vi "test_CCDSetAndGetGain.vi"   [LabVIEW 2023]
uses:
  <vilib>/JDP Science/JSONtext/Variant to JSON Text.vi
  <vilib>/JDP Science/JSONtext/Set Item.vi
  <vilib>/JDP Science/JSONtext/LVClass Serializer/JSONtext LVClass Serializer.lvclass
  Source/Classes/CCD/CCD.lvclass
  <vilib>/addons/_JKI Toolkits/Caraya/classes/Assert/Assert.lvclass
  <vilib>/addons/_JKI Toolkits/Caraya/classes/Test/Test.lvclass
  <vilib>/addons/_JKI Toolkits/Caraya/classes/Assert/Assert Equal Value and Type_Variant.vi
  <vilib>/addons/_JKI Toolkits/Caraya/classes/Assert/Assert Not Error.vi
types:
  T1 = enum16{"High Light", "Best Dynamic Range", "High Sensitivity"}
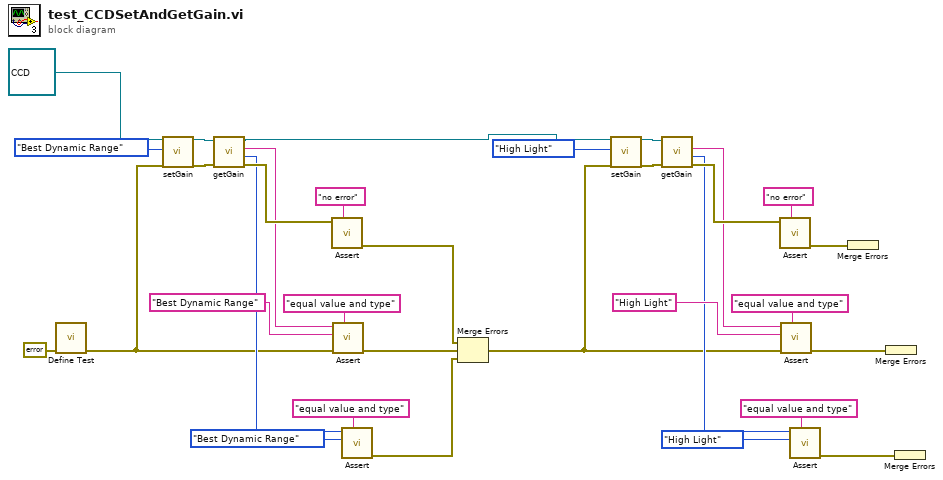
[diagram p0: block diagram]
diagram:
  n1 = call <vilib>:"Define Test.vi"("error in (no error)"=errorcluster {"status"=FALSE, "code"=0, "source"=""}) -> ("error out"=w7:errorcluster)  [unwired: 9 in, 1 out]
  n2 = call "setGain.vi"("CCD in"=refnum<class "CCD.lvclass"> refnum, "gain"=T1."Best Dynamic Range", "error in (no error)"=w7) -> ("CCD out"=w16:refnum<class "CCD.lvclass">, "error out"=w15:errorcluster)  [unwired: 11 in, 4 out]
  n3 = call "getGain.vi"("error in (no error)"=w15, "CCD in"=w16) -> ("error out"=w14:errorcluster, "gain token (enum)"=w8:T1, "gain info (string)"=w13:string, "CCD out"=w5:refnum<class "CCD.lvclass">)  [unwired: 6 in]
  n4 = call-poly <vilib>:"Assert.vi"("Label"="no error" ("Label (VI Title)"), "Not Error?"=w14) -> ("error out"=w3:errorcluster)  [unwired: 8 in, 1 out]
  n5 = call-poly <vilib>:"Assert.vi"("Label"="equal value and type" ("Label (VI Title)"), "error in (no error)"=w7, "Y"="Best Dynamic Range", "X"=w13) -> ("error out"=w2:errorcluster)  [unwired: 6 in, 1 out]
  n6 = call-poly <vilib>:"Assert.vi"("Label"="equal value and type" ("Label (VI Title)"), "Y"=T1."Best Dynamic Range" ("gain"), "X"=w8) -> ("error out"=w1:errorcluster)  [unwired: 7 in, 1 out]
  n7 = Merge Errors(w3, w2, w1) -> (w4:errorcluster)
  n8 = call "setGain.vi"("CCD in"=w5, "gain"=T1."High Light", "error in (no error)"=w4) -> ("CCD out"=w29:refnum<class "CCD.lvclass">, "error out"=w28:errorcluster)  [unwired: 11 in, 4 out]
  n9 = call "getGain.vi"("error in (no error)"=w28, "CCD in"=w29) -> ("error out"=w27:errorcluster, "gain token (enum)"=w20:T1, "gain info (string)"=w26:string)  [unwired: 6 in, 1 out]
  n10 = call-poly <vilib>:"Assert.vi"("Label"="no error" ("Label (VI Title)"), "Not Error?"=w27) -> ("error out"=w30:errorcluster)  [unwired: 8 in, 1 out]
  n11 = call-poly <vilib>:"Assert.vi"("Label"="equal value and type" ("Label (VI Title)"), "error in (no error)"=w4, "Y"="High Light", "X"=w26) -> ("error out"=w32:errorcluster)  [unwired: 6 in, 1 out]
  n12 = call-poly <vilib>:"Assert.vi"("Label"="equal value and type" ("Label (VI Title)"), "Y"=T1."High Light" ("gain"), "X"=w20) -> ("error out"=w22:errorcluster)  [unwired: 7 in, 1 out]
  n13 = Merge Errors(w30) -> ()  [unwired: 1 out]
  n14 = Merge Errors(w32) -> ()  [unwired: 1 out]
  n15 = Merge Errors(w22) -> ()  [unwired: 1 out]
